vi "Test Value In Tolerance.vi"(6 "Tolerance [%]":dbl, 10 "Value":dbl, 11 "Target":dbl) -> (3 "Within Tolerance":bool)   [LabVIEW 2020, in "Copy of Utility.lvlib"]
uses:
  Users/neilp/Desktop/Re-use Libraries/Utility/Copy of Utility.lvlib
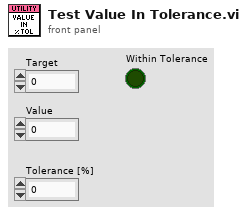
[diagram p1: front panel]
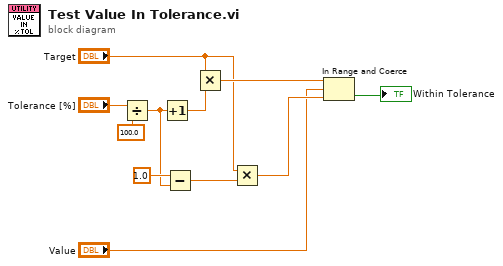
[diagram p0: block diagram]
diagram:
  n1 = Divide(x="Tolerance [%]", y=100.0) -> (x/y=w6:dbl)
  n2 = Increment(x=w6) -> (x+1=w9:dbl)
  n3 = Subtract(x=1.0, y=w6) -> (x-y=w5:dbl)
  n4 = Multiply(x="Target", y=w9) -> (x*y=w8:dbl)
  n5 = Multiply(x="Target", y=w5) -> (x*y=w3:dbl)
  n6 = In Range and Coerce(upper limit=w8, x="Value", lower limit=w3) -> (In Range?=→"Within Tolerance":bool)  [unwired: 1 out]
